vi "Fetch FPGA Data bkp.vi"(0 "Register Bus":T3, 1 "Tx Square Wave Generation":T2, 2 "Tx Sin Wave Generation":T1, 3 "Tx Constant":cluster{"cte I":i16, "cte Q":i16}, 4 "Beta":fxp<+,32,32>, 5 "error in":errorcluster, 6 "Select Wave":u8, 7 "vertical range [Vpp]":dbl=2.0 format="%#_6p", 8 "PRP (ms)":dbl, 9 "sample rate [S/s]":dbl=130000000.0 format="%#_6p", 10 "Pulse width (us)":dbl format="%#_10g", 11 "Guard width (us)":dbl format="%#_10g", 12 "Oversampling factor":u8, 13 "FPGA VI Reference In":refnum<k20>, 17 "nroCPI x CPI":u32, 18 "numRange":u32) -> (14 "Register Bus (out)":T3, 15 "Rx Waveform (CDB WDT)":waveform(cdb), 16 "Tx Waveform (CDB WDT)":waveform(cdb), 19 "error out":errorcluster)   [LabVIEW 2017]
doc: "Fetch Rx data from the device. It's required to call <b>Configure Stream</b> and <b>Initiate Stream</b> before calling this VI."
uses:
  <instrlib>/_niInstr/Register Bus/v0/Host/Public/Register Bus Session.ctl
  <instrlib>/_niInstr/Register Bus/v0/Host/Private/Session Data.ctl
  <vilib>/Utility/error.llb/Error Cluster From Error Code.vi
  <vilib>/rvi/errors/niLvFpgaAdjustHostInterfaceError.vi
  <vilib>/rvi/interface/nirviReadWriteControl/nirviReadWriteControl.xnode
  <vilib>/rvi/interface/nirviMethod/nirviMethod.xnode
  <instrlib>/_niInstr/Register Bus/v0/Host/niInstr Register Bus v0 Host.lvlib
  <vilib>/FPGAPlugInAG/Dynamic/niLvFpga_ReadFifo_Dynamic.vi
  <vilib>/rvi/errors/niLvFpgaMergeErrorWithErrorCode.vi
  NiFpgaLv.dll
  <vilib>/rvi/interface/Simulation/niFpgaSimulationCallBeginRW.vi
panel:
  out "normalization factor":fxp<+,8,1>
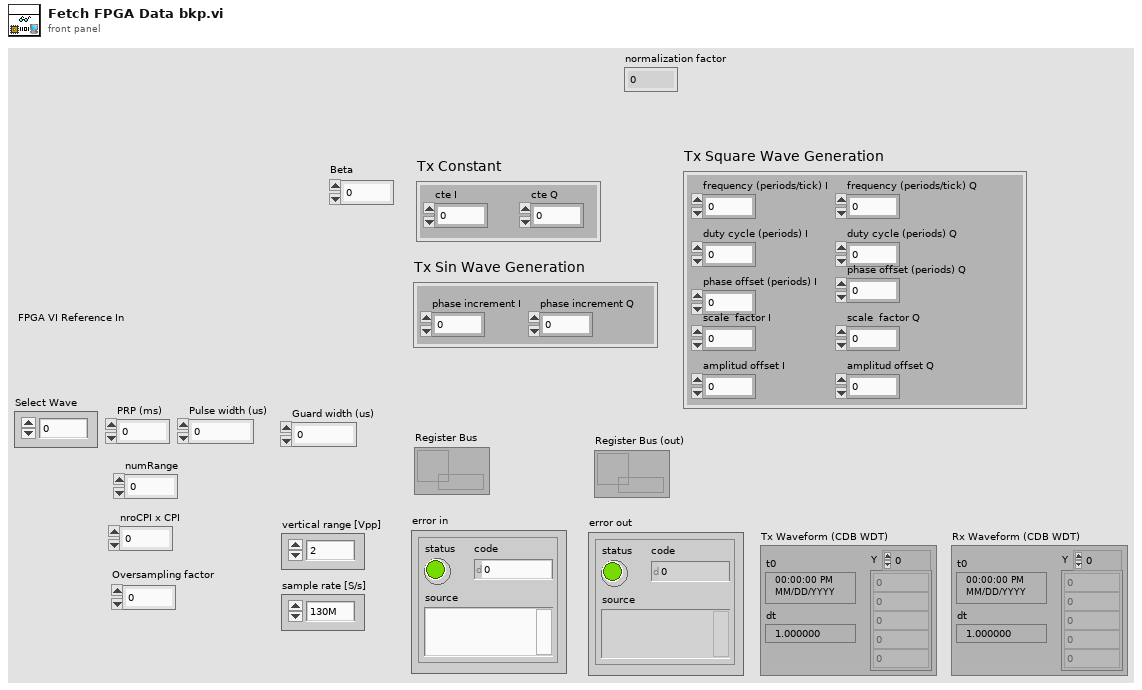
[diagram p1: front panel]
types:
  T1 = cluster{"phase increment":fxp<+/-,16,1>, "phase increment I":fxp<+/-,16,1>}
  T2 = cluster{"frequency (periods/tick) I":fxp<+,32,0>, "duty cycle (periods) I":fxp<+,32,0>, "phase offset (periods) I":fxp<+,32,0>, "frequency (periods/tick) Q":fxp<+,32,0>, "duty cycle (periods) Q":fxp<+,32,0>, "phase offset (periods) Q":fxp<+,32,0>, "scale  factor I":fxp<+/-,16,1>, "amplitud offset I":fxp<+/-,16,16>, "scale  factor Q":fxp<+/-,16,1>, "amplitud offset Q":fxp<+/-,16,16>}
  T3 = typedef "niInstr Register Bus v0 Host.lvlib/Register Bus Session.ctl" = refnum<queue>
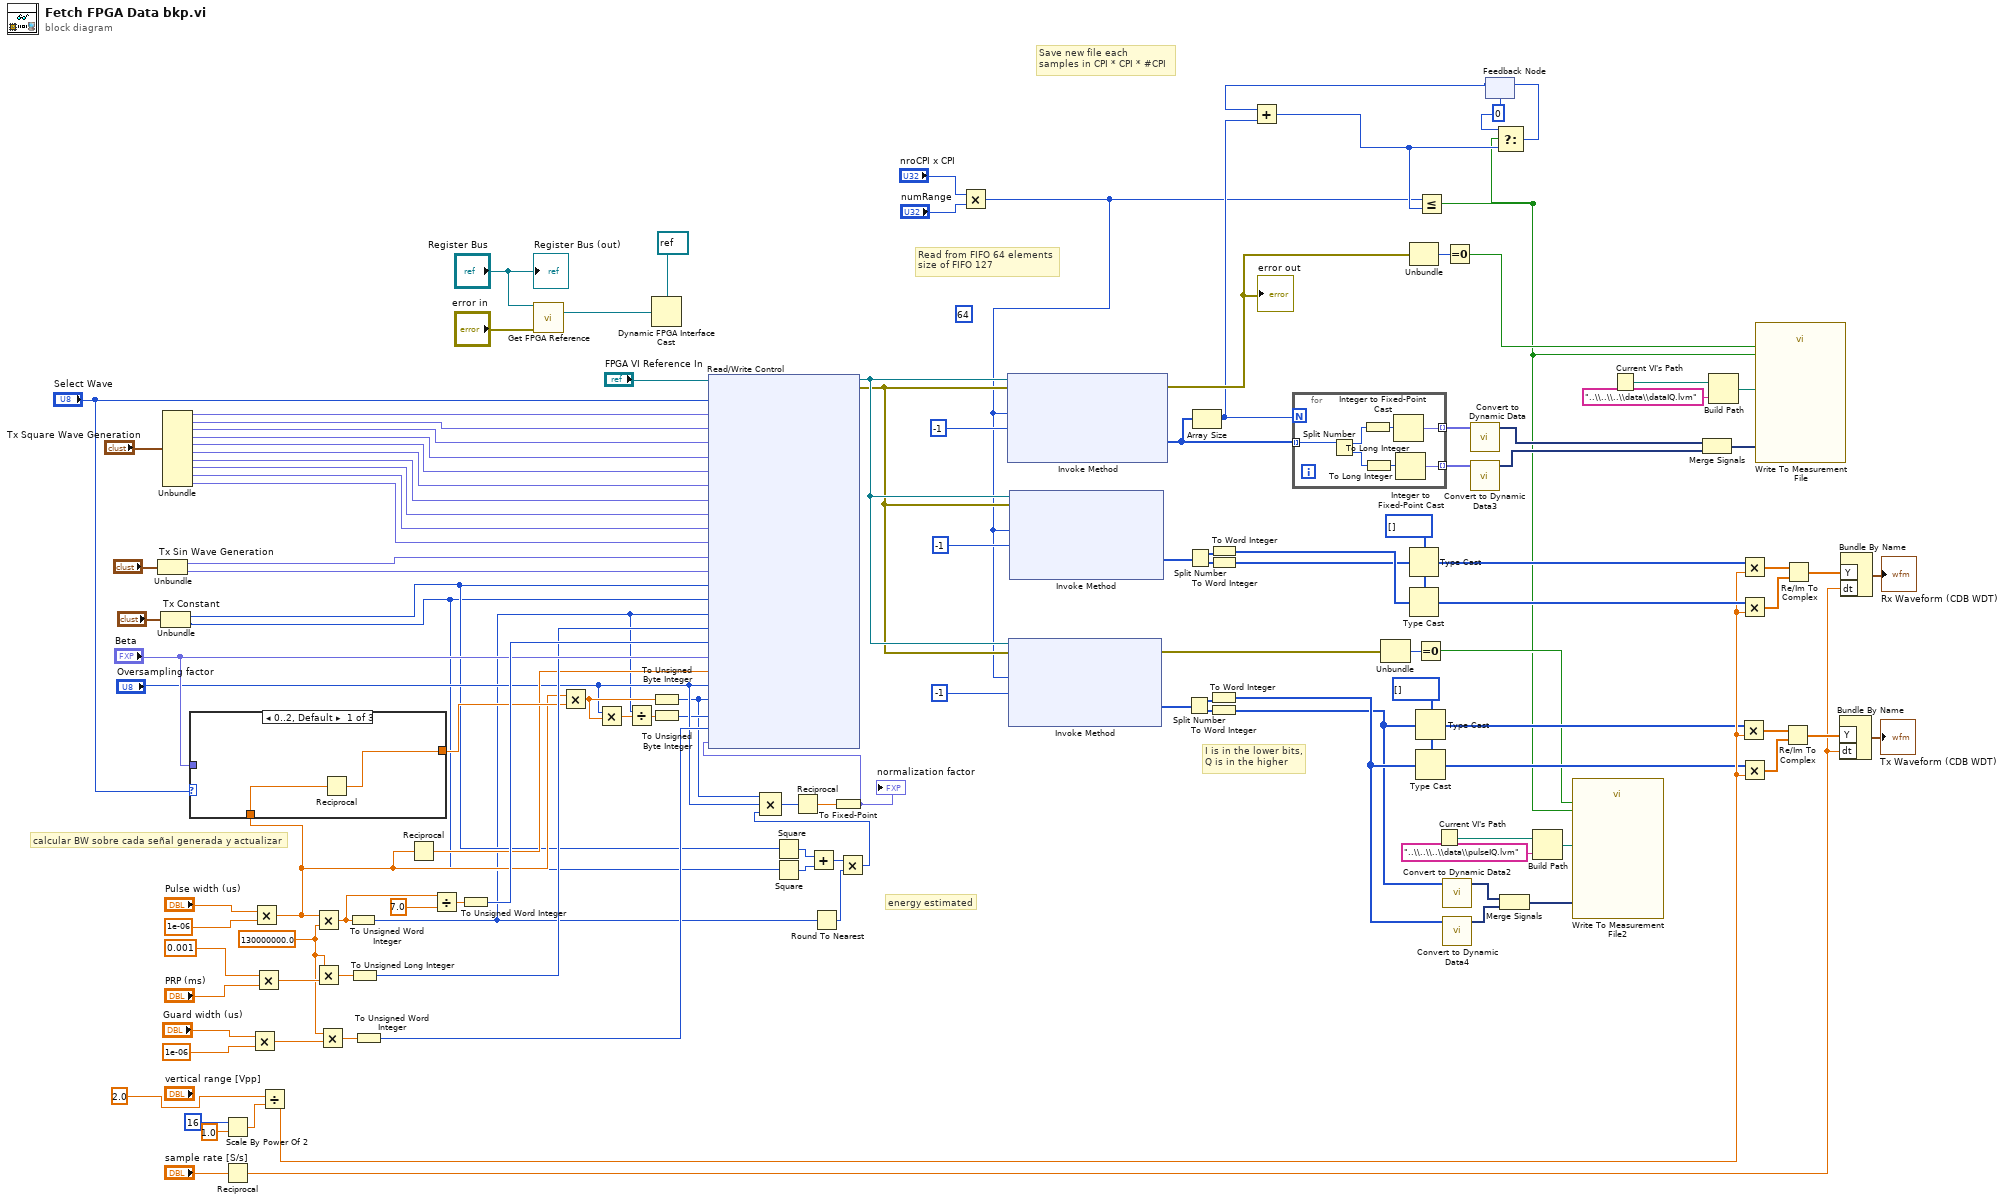
[diagram p0: block diagram]
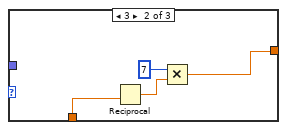
[diagram p2: hidden frame]
diagram:
  (unwired) u32 64 ("Number of Elements")
  w60 = u32 0
  w77 = i16[] []
  w28 = 130000000.0
  w120 = i16[] []
  # "I is in the lower bits,\nQ is in the higher"
  # "energy estimated"
  # "Read from FIFO 64 elements\nsize of FIFO 127"
  # "Save new file each \nsamples in CPI * CPI * #CPI"
  # "calcular BW sobre cada señal generada y actualizar"
  n1 = Unbundle("Tx Sin Wave Generation") -> ("phase increment"=w91:fxp<+/-,16,1>, "phase increment I"=w90:fxp<+/-,16,1>)
  n2 = Unbundle("Tx Constant") -> ("cte I"=w11:i16, "cte Q"=w10:i16)
  n3 = Unbundle("Tx Square Wave Generation") -> ("frequency (periods/tick) I"=w102:fxp<+,32,0>, "duty cycle (periods) I"=w101:fxp<+,32,0>, "phase offset (periods) I"=w100:fxp<+,32,0>, "frequency (periods/tick) Q"=w99:fxp<+,32,0>, "duty cycle (periods) Q"=w98:fxp<+,32,0>, "phase offset (periods) Q"=w97:fxp<+,32,0>, "scale  factor I"=w96:fxp<+/-,16,1>, "amplitud offset I"=w95:fxp<+/-,16,16>, "scale  factor Q"=w94:fxp<+/-,16,1>, "amplitud offset Q"=w93:fxp<+/-,16,16>)
  n4 = Scale By Power Of 2(n=i16 16 ("ADC Resolution (bits)"), x=1.0) -> (x*2^n=w121:dbl)
  n5 = Reciprocal(x="sample rate [S/s]") -> (1/x=w41:dbl)
  n6 = Multiply(x="Guard width (us)", y=1e-06) -> (x*y=w29:dbl)
  n7 = Multiply(x="Pulse width (us)", y=1e-06) -> (x*y=w39:dbl)
  n8 = case shown="0..2, Default" "Select Wave" {
    tunnel: w39 -> [w127 w129 _]
    tunnel: [w126 w130 w132] -> w40
    tunnel: "Beta" -> [_ _ w132]
    frame 0..2, Default {
      n9 = Reciprocal(x=w127) -> (1/x=w126:dbl)
    }
    frame 3 {
      n10 = Reciprocal(x=w129) -> (1/x=w128:dbl)
      n11 = Multiply(x=u16 7, y=w128) -> (x*y=w130:dbl)
    }
    frame 4 {
    }
  }
  n12 = Multiply(x=0.001, y="PRP (ms)") -> (x*y=w33:dbl)
  n13 = Divide(x=2.0, y=w121) -> (x/y=w73:dbl)
  n14 = Multiply(x=w39, y=w28) -> (x*y=w107:dbl)
  n15 = Multiply(x=w28, y=w33) -> (x*y=w110:dbl)
  n16 = Multiply(x=w28, y=w29) -> (x*y=w30:dbl)
  n17 = To Unsigned Word Integer(number=w107) -> (unsigned 16bit integer=w4:u16)
  n18 = To Unsigned Long Integer(number=w110) -> (unsigned 32bit integer=w42:u32)
  n19 = To Unsigned Word Integer(number=w30) -> (unsigned 16bit integer=w27:u16)
  n20 = Reciprocal(x=w39) -> (1/x=w38:dbl)
  n21 = Divide(x=w107, y=7.0) -> (x/y=w108:dbl)
  n22 = To Unsigned Word Integer(number=w108) -> (unsigned 16bit integer=w104:u16)
  n23 = call <instrlib>:"Get FPGA Reference.vi"("session in"="Register Bus", "error in"="error in") -> ("fpga ref"=w112:refnum<k20>)  [unwired: 11 in, 2 out]
  n24 = Multiply(x=w39, y=w40) -> (x*y=w43:dbl)
  n25 = Multiply(x="Oversampling factor", y=w43) -> (x*y=w45:dbl)
  n26 = Divide(x=w4, y=w45) -> (x/y=w44:dbl)
  n27 = Dynamic FPGA Interface Cast(Session In=refnum<k20> refnum ("FPGA Interface"), Type=w112) -> ()  [unwired: 1 out]
  n28 = To Unsigned Byte Integer(number=w43) -> (unsigned 8bit integer=w16:u8)
  n29 = To Unsigned Byte Integer(number=w44) -> (unsigned 8bit integer=w25:u8)
  n30 = Square(x=w11) -> (x^2=w8:u32)
  n31 = Square(x=w10) -> (x^2=w9:u32)
  n32 = Add(x=w8, y=w9) -> (x+y=w7:u32)
  n33 = Round To Nearest(number=w4) -> (nearest integer value=w6:u16)
  n34 = Multiply(x=w7, y=w6) -> (x*y=w5:u32)
  n35 = Compound Arithmetic op=MULTIPLY(w16, "Oversampling factor", w5) -> (w24:u32)
  n36 = Reciprocal(x=w24) -> (1/x=w15:dbl)
  n37 = To Fixed-Point(number=w15) -> (fixed-point=w17:fxp<+,38,0>)  [unwired: 1 in]
  "normalization factor" <- w17
  n38 = xnode "Read/Write Control"("FPGA VI Reference In"="FPGA VI Reference In", "Select Wave"="Select Wave", "frequency (periods/tick) I"=w102, "duty cycle (periods) I"=w101, "phase offset (periods) I"=w100, "scale  factor I"=w99, "amplitud offset I"=w98, "frequency (periods/tick) Q"=w97, "duty cycle (periods) Q"=w96, "scale  factor Q"=w95, "amplitud offset Q"=w94, "phase offset (periods) Q"=w93, "phase increment I"=w91, "phase increment Q"=w90, "cte I"=w11, "cte Q"=w10, "Pulse width"=w4, "PRP"=w42, "Barker width"=w104, "Beta"="Beta", "1/tao"=w38, "Oversampling factor"="Oversampling factor", "BW*tao"=w16, "Sampling width"=w25, "Guard width"=w27, "Normalization factor"=w17) -> ("FPGA VI Reference Out"=w75:refnum<k20>, "error out"=w74:errorcluster)  [unwired: 1 in]
  n39 = Multiply(x="nroCPI x CPI", y="numRange") -> (x*y=w3:u32)
  n40 = xnode "Invoke Method"("FPGA VI Reference In"=w75, "error in"=w74, "Number of Elements"=w3, "Timeout (ms)"=-1) -> ("error out"=w65:errorcluster, "Data"=w13:u64[])  [unwired: 2 out]
  "error out" <- w65
  n41 = xnode "Invoke Method"("FPGA VI Reference In"=w75, "error in"=w74, "Number of Elements"=w3, "Timeout (ms)"=-1) -> ("error out"=w62:errorcluster, "Data"=w2:u32[])  [unwired: 2 out]
  n42 = xnode "Invoke Method"("FPGA VI Reference In"=w75, "error in"=w74, "Number of Elements"=w3, "Timeout (ms)"=-1) -> ("Data"=w82:u32[])  [unwired: 3 out]
  n43 = Split Number(x=w2) -> (hi(x)=w51:u16[], lo(x)=w49:u16[])
  n44 = Split Number(x=w82) -> (hi(x)=w55:u16[], lo(x)=w53:u16[])
  n45 = Array Size(array=w13) -> (size(s)=w36:i32)
  n46 = To Word Integer(number=w51) -> (16bit integer=w50:i16[])
  n47 = To Word Integer(number=w49) -> (16bit integer=w48:i16[])
  n48 = To Word Integer(number=w55) -> (16bit integer=w54:i16[])
  n49 = To Word Integer(number=w53) -> (16bit integer=w52:i16[])
  n50 = for {
    N: w36 -> [_]
    tunnel: w13 -> [w135] mode=indexing
    tunnel: [w136] -> w35 mode=indexing
    tunnel: [w133] -> w34 mode=indexing
    n51 = Split Number(x=w135) -> (hi(x)=w139:u32, lo(x)=w138:u32)
    n52 = To Long Integer(number=w139) -> (32bit integer=w137:i32)
    n53 = To Long Integer(number=w138) -> (32bit integer=w134:i32)
    n54 = Integer to Fixed-Point Cast(integer=w137) -> (fixed-point=w136:fxp<+/-,32,8>)  [unwired: 1 in]
    n55 = Integer to Fixed-Point Cast(integer=w134) -> (fixed-point=w133:fxp<+/-,32,8>)  [unwired: 1 in]
  }
  n56 = Unbundle(w62) -> ("code"=w63:i32)  [unwired: 2 out]
  n57 = Unbundle(w65) -> ("code"=w66:i32)  [unwired: 2 out]
  n58 = Type Cast(type=w120, x=w52) -> (*(type *) &x=w119:i16[])
  n59 = Type Cast(type=w120, x=w54) -> (*(type *) &x=w118:i16[])
  n60 = Equal To 0?(x=w63) -> (x = 0?=w61:bool)
  n61 = Type Cast(type=w77, x=w48) -> (*(type *) &x=w69:i16[])
  n62 = Type Cast(type=w77, x=w50) -> (*(type *) &x=w68:i16[])
  n63 = Current VI's Path() -> (path=w19:path)
  n64 = call "Convert to Dynamic Data2"("Array"=w48) -> ("Dynamic Data Type"=w71:dynamicdata)  [unwired: 3 in]
  n65 = call "Convert to Dynamic Data4"("Array"=w50) -> ("Dynamic Data Type"=w70:dynamicdata)  [unwired: 3 in]
  n66 = Equal To 0?(x=w66) -> (x = 0?=w64:bool)
  n67 = call "Convert to Dynamic Data"("Array"=w35) -> ("Dynamic Data Type"=w37:dynamicdata)  [unwired: 3 in]
  n68 = call "Convert to Dynamic Data3"("Array"=w34) -> ("Dynamic Data Type"=w72:dynamicdata)  [unwired: 3 in]
  n69 = feedback #1(w60) -> (w58:u32)
  n70 = Add(x=w58, y=w36) -> (x+y=w57:u32)
  n71 = Less Or Equal?(x=w3, y=w57) -> (x <= y?=w1:bool)
  n72 = Select(t=w60, s=w1, f=w57) -> (s? t:f=w59:u32)
  n73 = feedback-in #1(w59) -> ()
  n74 = Merge Signals(w71, w70) -> (w67:dynamicdata)
  n75 = Build Path(base path=w19, name or relative path="..\\..\\..\\data\\pulseIQ.lvm") -> (appended path=w18:path)
  n76 = call "Write To Measurement File2"("Signals"=w67, "Enable"=w61, "new_file"=w1, "Filename"=w18) -> ()  [unwired: 13 in, 3 out]
  n77 = Current VI's Path() -> (path=w22:path)
  n78 = Merge Signals(w37, w72) -> (w12:dynamicdata)
  n79 = Build Path(base path=w22, name or relative path="..\\..\\..\\data\\dataIQ.lvm") -> (appended path=w21:path)
  n80 = Multiply(x=w69, y=w73) -> (x*y=w78:dbl[])
  n81 = Multiply(x=w119, y=w73) -> (x*y=w117:dbl[])
  n82 = Multiply(x=w68, y=w73) -> (x*y=w79:dbl[])
  n83 = Multiply(x=w118, y=w73) -> (x*y=w116:dbl[])
  n84 = call "Write To Measurement File"("Signals"=w12, "Enable"=w64, "new_file"=w1, "Filename"=w21) -> ()  [unwired: 13 in, 3 out]
  n85 = Re/Im To Complex(1:w79, 2:w78) -> (0:w80:cdb[])
  n86 = Re/Im To Complex(1:w116, 2:w117) -> (0:w115:cdb[])
  n87 = Bundle By Name("Y"=w80, "dt"=w41) -> (→"Tx Waveform (CDB WDT)":waveform(cdb))  [unwired: 1 in]
  n88 = Bundle By Name("Y"=w115, "dt"=w41) -> (→"Rx Waveform (CDB WDT)":waveform(cdb))  [unwired: 1 in]
  "Register Bus (out)" <- "Register Bus"
